vi "_PC_Pub_FM closeFile.vi"(8 "error in (no error)":errorcluster, 11 "FM in":refnum<class "FM.lvclass">) -> (0 "error out":errorcluster, 2 "filePath":path, 3 "FM out":refnum<class "FM.lvclass">)   [LabVIEW 2018, in "FM.lvclass"]
uses:
  FM.lvclass
  FM.lvclass/FM.ctl
  TDMSAdv.lvclass
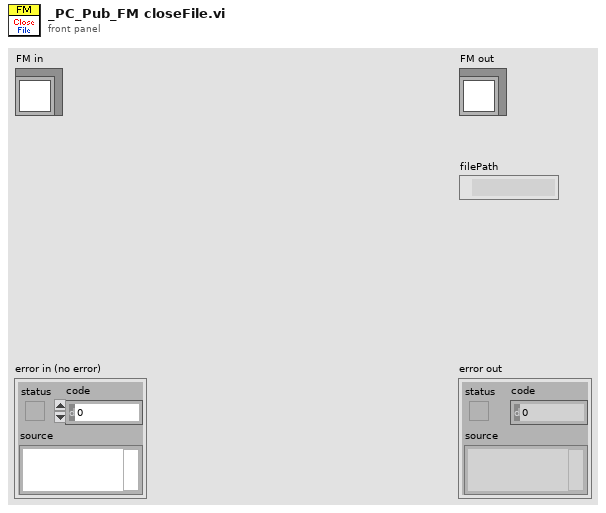
[diagram p1: front panel]
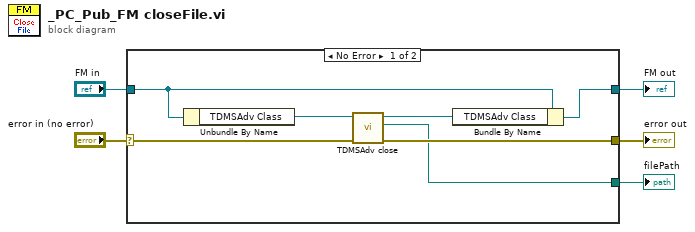
[diagram p0: block diagram]
diagram:
  n1 = case shown="No Error" "error in (no error)" {
    selector: "error in (no error)" -> [w12 w14]
    tunnel: [w7 w14] -> w4
    tunnel: [w9 w13] -> w2
    tunnel: "FM in" -> [w10 w13]
    tunnel: [w6 _] -> w1
    frame No Error {
      n2 = Unbundle By Name(w10) -> ("TDMSAdv Class"=w11:refnum<class "TDMSAdv.lvclass">)
      n3 = call "TDMSAdv close.vi"("error in (no error)"=w12, "TDMSAdv in"=w11) -> ("error out"=w7:errorcluster, "filePath"=w6:path, "TDMSAdv out"=w8:refnum<class "TDMSAdv.lvclass">)  [unwired: 7 in]
      n4 = Bundle By Name(cluster=w10, "TDMSAdv Class"=w8) -> (w9:refnum<class "FM.lvclass">)
    }
    frame Error {
    }
  }
  "error out" <- w4
  "FM out" <- w2
  "filePath" <- w1
